vi "MILStateFeedbackControllerX.vi"(0 "Ac":dbl[](array[numeric])=[0.0, 0.0, 0.0, 0.0], 1 "DispX":dbl, 3 "P1X":dbl, 6 "DispY":dbl, 7 "Bc":dbl[](array[numeric])=[0.0, 0.0, 0.0, 0.0], 9 "Cc":dbl[](array[numeric])=[1.0, 0.0], 10 "ForceY":dbl, 11 "Dc":dbl[](array[numeric])=[0.0, 0.0], 12 "ForceX":dbl, 14 "P2X":dbl) -> (4 "ValveCMDX":dbl, 15 "ValveCMDY":dbl)   [LabVIEW 2020]
uses:
  <vilib>/Analysis/NI_AALBase.lvlib
  <vilib>/Analysis/baseanly.llb/A x Vector.vi
  <vilib>/Analysis/NI_AALBLAS.lvlib
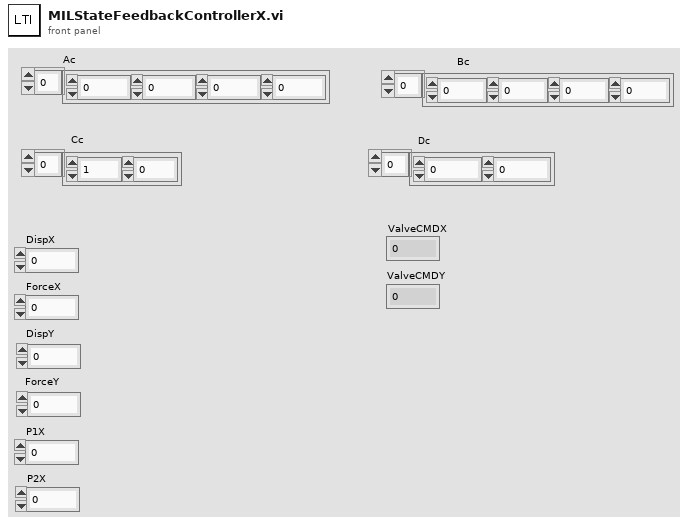
[diagram p1: front panel]
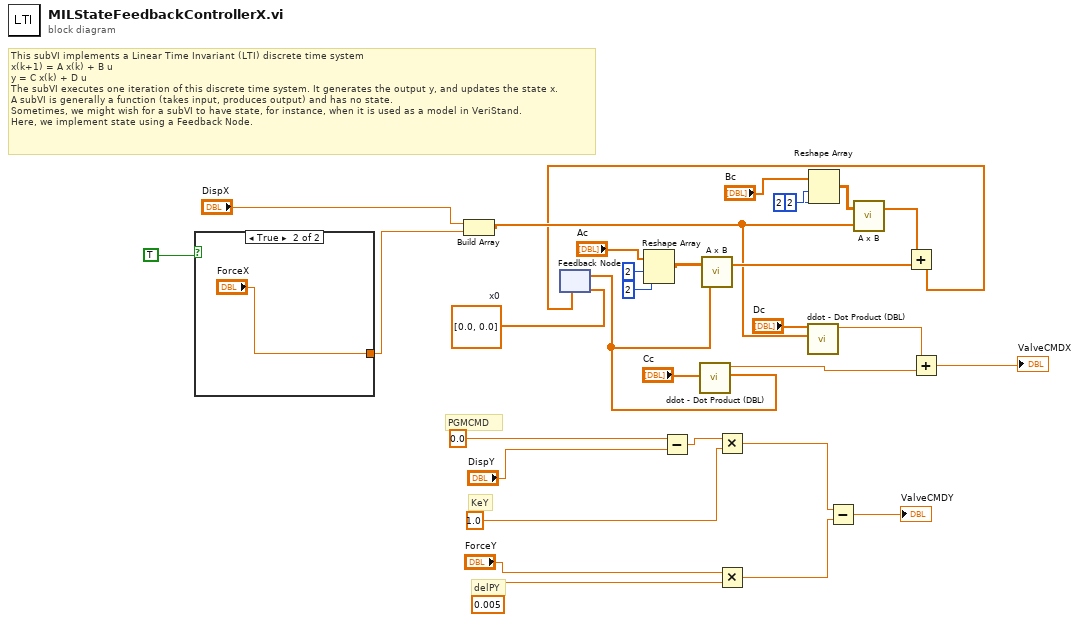
[diagram p0: block diagram]
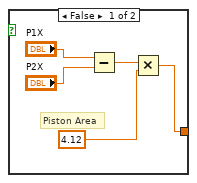
[diagram p2: hidden frame]
diagram:
  w31 = dbl[] [0.0, 0.0]  # x0
  # "PGMCMD"
  # "delPY"
  # "KeY"
  # "This subVI implements a Linear Time Invariant (LTI) discrete time system\nx(k+1) = A x(k) + B u\ny = C x(k) + D u\nThe subVI executes one iteration of this discrete time system. It generates the output y, and updates the state x.\nA subVI is generally a function (takes input, produces output) and has no state.\nSometimes, we might wish for a subVI to have state, for instance, when it is used as a model in VeriStand.\nHere, we implement state using a Feedback Node."
  n1 = case shown="True" TRUE {
    tunnel: [w32 "ForceX"] -> w12
    frame False {
      # "Piston Area"
      n2 = Subtract(x="P1X", y="P2X") -> (x-y=w36:dbl)
      n3 = Multiply(x=w36, y=4.12) -> (x*y=w32:dbl)
    }
    frame True {
    }
  }
  n4 = Build Array("DispX", w12) -> (w11:dbl[])
  n5 = feedback #1(w31) -> (w29:dbl[])
  n6 = Reshape Array("Ac", 2 ("dimension size"), 2 ("dimension size")) -> (w7:dbl[][])
  n7 = Subtract(x=0.0 ("PGMCMDY"), y="DispY") -> (x-y=w21:dbl)
  n8 = call <vilib>:"ddot - Dot Product (DBL).vi"("y"=w29, "x"="Cc") -> ("ddot"=w28:dbl)  [unwired: 8 in, 1 out]
  n9 = call-poly <vilib>:"A x B.vi"("Vector"=w29, "A"=w7) -> ("A x Vector"=w30:dbl[])  [unwired: 1 out]
  n10 = Multiply(x=w21, y=1.0 ("KeY")) -> (x*y=w17:dbl)
  n11 = Multiply(x="ForceY", y=0.005 ("delPY")) -> (x*y=w16:dbl)
  n12 = call <vilib>:"ddot - Dot Product (DBL).vi"("y"=w11, "x"="Dc") -> ("ddot"=w25:dbl)  [unwired: 8 in, 1 out]
  n13 = Reshape Array("Bc", 2 ("dimension size"), 2 ("dimension size")) -> (w3:dbl[][])
  n14 = Subtract(x=w17, y=w16) -> (x-y=→"ValveCMDY":dbl)
  n15 = call-poly <vilib>:"A x B.vi"("Vector"=w11, "A"=w3) -> ("A x Vector"=w27:dbl[])  [unwired: 1 out]
  n16 = Add(x=w27, y=w30) -> (x+y=w1:dbl[])
  n17 = feedback-in #1(w1) -> ()
  n18 = Add(x=w25, y=w28) -> (x+y=→"ValveCMDX":dbl)
